vi "Get Configuration.vi"(8 "error in (no error)":errorcluster, 11 "IO-4 Bricklet in":refnum<class "IO-4 Bricklet.lvclass">) -> (0 "error out":errorcluster, 1 "Value Mask":u8, 2 "Direction Mask":u8, 3 "IO-4 Bricklet out":refnum<class "IO-4 Bricklet.lvclass">)   [LabVIEW 2011, in "Tinkerforge.lvlib" / "IO-4 Bricklet.lvclass"]
doc: "Returns a value bit mask and a direction bit mask.\n\nFor example: A return value of the bitstrings “1100” and “1010” for direction and value means that:\n\n pin 0 is configured as input pull up,\n pin 1 is configured as input default,\n pin 2 is configured as output high\n and pin 3 is are configured as output low."
uses:
  IO-4 Bricklet.lvclass
  Type Definitions/Configuration.ctl
  Device/Device.lvclass
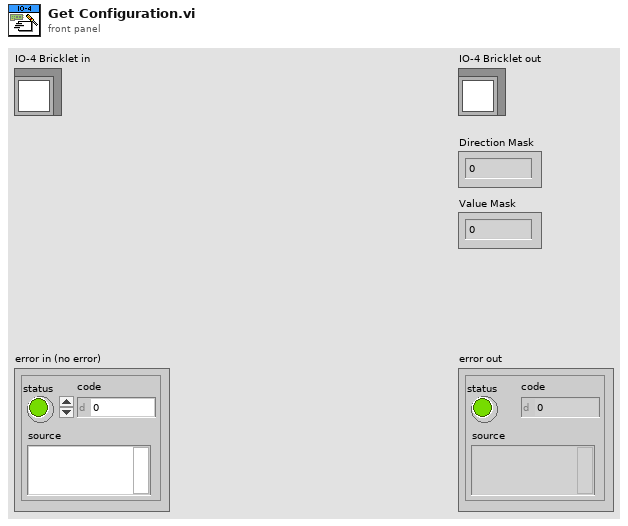
[diagram p1: front panel]
types:
  T1 = typedef "Tinkerforge.lvlib/IO-4 Bricklet.lvclass/Configuration.ctl" = cluster{"Direction Mask":u8, "Value Mask":u8}
  T2 = typedef "Tinkerforge.lvlib/IP Connection.lvclass/Answer.ctl" = cluster{"Request GUID":string, "Request Type":T3, "Sucessful":bool, "Data":variant, "Error":errorcluster}
  T3 = typedef "Tinkerforge.lvlib/IP Connection.lvclass/Request Type.ctl" = enum8{"Invalid", "Write"}
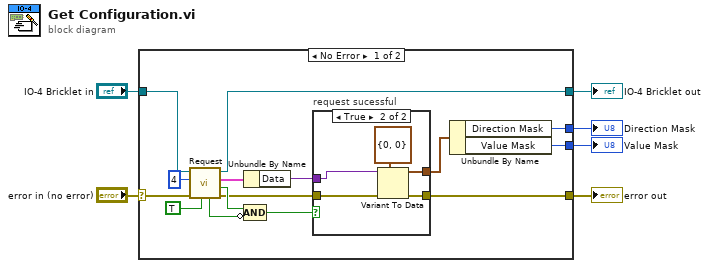
[diagram p0: block diagram]
diagram:
  n1 = case shown="No Error" "error in (no error)" {
    selector: "error in (no error)" -> [w21 w29]
    tunnel: [w10 w29] -> w5
    tunnel: [w19 w28] -> w3
    tunnel: "IO-4 Bricklet in" -> [w20 w28]
    tunnel: [w8 _] -> w2
    tunnel: [w7 _] -> w1
    frame No Error {
      n2 = call "Request.vi"("Response"=TRUE, "error in (no error)"=w21, "Function ID"=u8 4, "Device in"=w20) -> ("error out"=w13:errorcluster, "Sucessful"=w15:bool, "Answer"=w12:T2, "Device out"=w19:refnum<class "IO-4 Bricklet.lvclass">, "timed out"=w16:bool)  [unwired: 3 in]
      n3 = Unbundle By Name(w12) -> ("Data"=w11:variant)
      n4 = Compound Arithmetic op=AND(w15, invert w16) -> (w14:bool)
      n5 = case "request sucessful" shown="True" w14 {
        tunnel: w13 -> [w22 w27]
        tunnel: w11 -> [_ w25]
        tunnel: [_ w24] -> w9
        tunnel: [w22 w23] -> w10
        frame False {
        }
        frame True {
          n6 = Variant To Data(error in=w27, type=T1 {"Direction Mask"=0, "Value Mask"=0}, Variant=w25) -> (data=w24:T1, error out=w23:errorcluster)
        }
      }
      n7 = Unbundle By Name(w9) -> ("Direction Mask"=w8:u8, "Value Mask"=w7:u8)
    }
    frame Error {
    }
  }
  "error out" <- w5
  "IO-4 Bricklet out" <- w3
  "Direction Mask" <- w2
  "Value Mask" <- w1
